vi "Gamepad NanoDrive Control.vi"(1 "handle":i32) -> ()   [LabVIEW 2012]
uses:
  <vilib>/Utility/miscctls.llb/LVPointTypeDef.ctl
  <vilib>/Utility/file.llb/Read From Spreadsheet File (I64).vi
  <vilib>/Utility/inputDevices.llb/joystickAcquire.vi
  <vilib>/Utility/inputDevices.llb/closeJoystick.vi
  Madlib.dll
panel:
  out "Y axis":dbl
  out "X axis":dbl
  out "yRead":dbl=5.0 step=0.1 format="%.3f"
  out "xRead":dbl=5.0 step=0.1 format="%.3f"
  in  "left":bool
  in  "down":bool
  in  "right":bool
  in  "up":bool
  in  "closed?":bool
  in  "Slide":cluster{u32, u32}(slide)={0, 5} scale=0.0..7.0
  in  "configure":bool
  out "button selection refs":T1
  in  "yf":u16(ring)=4 items=["1 X"=1, "2 A"=2, "3 B"=3, "4 Y"=4, "5 LB"=5, "6 RB"=6, "7 LT"=7, "8 RT"=8, "9 Back"=9]
  in  "xf":u16(ring)=3 items=["1 X"=1, "2 A"=2, "3 B"=3, "4 Y"=4, "5 LB"=5, "6 RB"=6, "7 LT"=7, "8 RT"=8, "9 Back"=9]
  in  "yf xr 2":u16(ring)=5 items=["1 X"=1, "2 A"=2, "3 B"=3, "4 Y"=4, "5 LB"=5, "6 RB"=6, "7 LT"=7, "8 RT"=8, "9 Back"=9]
  in  "halt 3":u16(ring)=9 items=["1 X"=1, "2 A"=2, "3 B"=3, "4 Y"=4, "5 LB"=5, "6 RB"=6, "7 LT"=7, "8 RT"=8, "9 Back"=9]
  in  "yf xf 2":u16(ring)=6 items=["1 X"=1, "2 A"=2, "3 B"=3, "4 Y"=4, "5 LB"=5, "6 RB"=6, "7 LT"=7, "8 RT"=8, "9 Back"=9]
  in  "yr xr 2":u16(ring)=7 items=["1 X"=1, "2 A"=2, "3 B"=3, "4 Y"=4, "5 LB"=5, "6 RB"=6, "7 LT"=7, "8 RT"=8, "9 Back"=9]
  in  "yr":u16(ring)=2 items=["1 X"=1, "2 A"=2, "3 B"=3, "4 Y"=4, "5 LB"=5, "6 RB"=6, "7 LT"=7, "8 RT"=8, "9 Back"=9]
  in  "yr xf 2":u16(ring)=8 items=["1 X"=1, "2 A"=2, "3 B"=3, "4 Y"=4, "5 LB"=5, "6 RB"=6, "7 LT"=7, "8 RT"=8, "9 Back"=9]
  in  "xr":u16(ring)=1 items=["1 X"=1, "2 A"=2, "3 B"=3, "4 Y"=4, "5 LB"=5, "6 RB"=6, "7 LT"=7, "8 RT"=8, "9 Back"=9]
  in  "down-left":bool
  in  "down-right":bool
  in  "up-left":bool
  in  "up-right":bool
  in  "yStep":dbl=1.0 min=0.01905 max=4.0 format="%.3f"
  in  "xStep":dbl=1.0 min=0.01905 max=4.0 format="%.3f"
  in  "Invert":bool=TRUE
  in  "Invert":bool
  # "Single Step Controls"
  # "Position"
  # "Step distance"
  # "Current position"
  # "X axis"
  # "X axis"
  # "um"
  # "um"
  # "Y axis"
  # "Y axis"
  # "um"
  # "um"
  # "Step"
  # "Commanded position"
  # "um"
  # "um"
  # "Configuration"
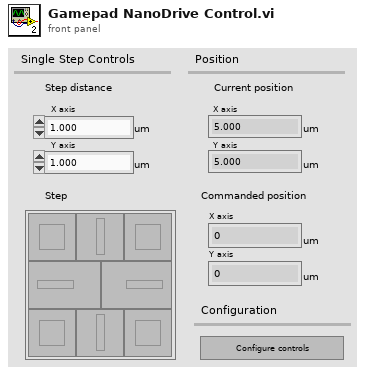
[diagram p1: front panel]
types:
  T1 = cluster{"xr":refnum<vi>, "yr":refnum<vi>, "xf":refnum<vi>, "yf":refnum<vi>, "yf xr 2":refnum<vi>, "yf xf 2":refnum<vi>, "yr xr 2":refnum<vi>, "yr xf 2":refnum<vi>, "halt 2":refnum<vi>}
  T2 = enum16{"open", "replace", "create", "open or create", "replace or create", "replace or create with confirmation"}
  T3 = typedef "LVPointTypeDef.ctl" = cluster{"Horizontal":i16, "Vertical":i16}
  T4 = cluster{"Controls":cluster{"Commands":cluster{"unused":bool}, "Values":cluster{"up":u16, "right":u16}}, "ControlRefs":cluster{"Commands":cluster{"unused":refnum<vi>}, "Values":cluster{"up":refnum<vi>, "right":refnum<vi>}}, "Variables":cluster{"Commands":cluster{"up_changed":bool, "right_changed":bool}, "Values":cluster{"unused":i32}}}
  T5 = cluster{"Controls":cluster{"Commands":cluster{"right":bool, "left":bool, "up":bool, "down":bool, "down-left":bool, "up-left":bool, "up-right":bool, "down-right":bool}, "Values":cluster{"xStep":dbl, "yStep":dbl, "xRead":dbl, "yRead":dbl}}, "ControlRefs":cluster{"Commands":cluster{"right":refnum<vi>, "left":refnum<vi>, "up":refnum<vi>, "down":refnum<vi>, "down-left":refnum<vi>, "up-left":refnum<vi>, "up-right":refnum<vi>, "down-right":refnum<vi>}, "Values":cluster{"X step":refnum<vi>, "Y step":refnum<vi>, "xRead":refnum<vi>, "yRead":refnum<vi>}}, "Variables":cluster{"Commands":cluster{"unused":bool}, "Values":cluster{"xCommand":dbl, "yCommand":dbl, "xCalibration":dbl, "yCalibration":dbl}}}
  T6 = cluster{"xr":refnum<vi>, "yr":refnum<vi>, "xf":refnum<vi>, "yf":refnum<vi>, "yf xr 2":refnum<vi>, "yf xf 2":refnum<vi>, "yr xr 2":refnum<vi>, "yr xf 2":refnum<vi>, "halt 3":refnum<vi>}
  T7 = cluster{"X axis":i32, "Y axis":i32, "Z axis":i32, "X axis rotation":i32, "Y axis rotation":i32, "Z axis rotation":i32, "U axis":i32, "V axis":i32}
  T8 = cluster{"button 1":bool, "button 2":bool, "button 3":bool, "button 4":bool, "button 5":bool, "button 6":bool, "button 7":bool, "button 8":bool, "button 9":bool, "button 10":bool, "button 11":bool, "button 12":bool, "button 13":bool, "button 14":bool, "button 15":bool, "button 16":bool, "button 17":bool, "button 18":bool, "button 19":bool, "button 20":bool, "button 21":bool, "button 22":bool, "button 23":bool, "button 24":bool, "button 25":bool, "button 26":bool, "button 27":bool, "button 28":bool, "button 29":bool, "button 30":bool, "button 31":bool, "button 32":bool}
  T9 = cluster{"left":bool, "down":bool, "right":bool, "up":bool, "up-left":bool, "up-right":bool, "down-left":bool, "down-right":bool, "halt":bool, "button 10":bool}
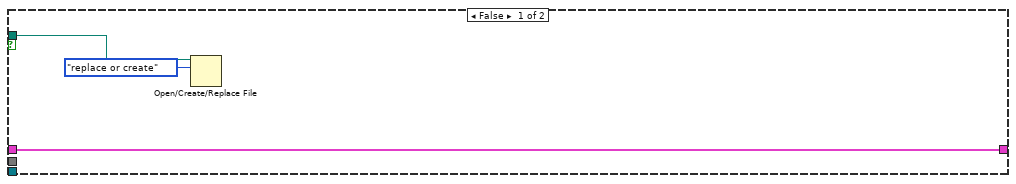
[diagram p2: hidden frame]
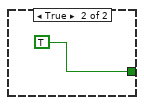
[diagram p4: hidden frame]
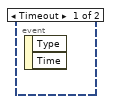
[diagram p9: hidden frame]
diagram:
  n1 = flat-sequence {
    tunnel: [w54] -> w39
    tunnel: [w53] -> w38
    tunnel: [w52] -> w37
    tunnel: [w71] -> w32
    tunnel: [w70] -> w31
    tunnel: [w69] -> w30
    tunnel: w39 -> [w71]
    tunnel: w38 -> [w66]
    tunnel: w37 -> [w69]
    tunnel: w32 -> [w74]
    tunnel: [w73] -> w41
    tunnel: w31 -> [w84]
    tunnel: [w84] -> w40
    tunnel: w30 -> [w72]
    tunnel: [w72] -> w36
    tunnel: w41 -> [w90]
    tunnel: [w90] -> w43
    tunnel: w40 -> [w96]
    tunnel: [w96] -> w42
    tunnel: w36 -> [w87]
    tunnel: [w86] -> w34
    tunnel: [w145] -> w47
    tunnel: [w146] -> w45
    tunnel: w42 -> [w146]
    tunnel: w43 -> [w145]
    tunnel: [w138] -> w35
    tunnel: w34 -> [w138]
    tunnel: [w151] -> w15
    tunnel: [w150] -> w13
    tunnel: w47 -> [w149]
    tunnel: [w149] -> w11
    tunnel: [w148] -> w9
    tunnel: w45 -> [w148]
    tunnel: [w147] -> w7
    tunnel: w35 -> [w147]
    tunnel: w15 -> [w176]
    tunnel: [w176] -> w14
    tunnel: w13 -> [w175]
    tunnel: [w175] -> w12
    tunnel: w11 -> [w174]
    tunnel: [w174] -> w10
    tunnel: w9 -> [w173]
    tunnel: [w173] -> w8
    tunnel: w7 -> [w172]
    tunnel: [w172] -> w6
    tunnel: ["handle"] -> w5
    tunnel: [w183] -> w27
    tunnel: [w184] -> w25
    tunnel: [w182] -> w23
    tunnel: w14 -> [w184]
    tunnel: w12 -> [w183]
    tunnel: w10 -> [w181]
    tunnel: [w181] -> w21
    tunnel: w8 -> [w180]
    tunnel: [w180] -> w19
    tunnel: w6 -> [w179]
    tunnel: [w179] -> w17
    tunnel: w5 -> [w178]
    tunnel: [w177] -> w4
    tunnel: w27 -> [w211]
    tunnel: [w211] -> w26
    tunnel: w25 -> [w210]
    tunnel: [w210] -> w24
    tunnel: w23 -> [w206]
    tunnel: [w206] -> w22
    tunnel: w21 -> [w205]
    tunnel: [w205] -> w20
    tunnel: w19 -> [w204]
    tunnel: [w201] -> w18
    tunnel: w17 -> [w209]
    tunnel: [w209] -> w16
    tunnel: w4 -> [w200]
    tunnel: [w200] -> w2
    tunnel: w26 -> [w219]
    tunnel: [w219] -> w51
    tunnel: w24 -> [w220]
    tunnel: [w220] -> w50
    tunnel: w22 -> [w218]
    tunnel: [w218] -> w49
    tunnel: [u32 0 ("current button state")] -> w48
    tunnel: [w215] -> w46
    tunnel: w20 -> [w215]
    tunnel: [w214] -> w44
    tunnel: w18 -> [w214]
    tunnel: [w213] -> w33
    tunnel: w16 -> [w213]
    tunnel: [w212] -> w3
    tunnel: w2 -> [w212]
    tunnel: w49 -> [w229]
    tunnel: w50 -> [w231]
    tunnel: w51 -> [w230]
    tunnel: w48 -> [w228]
    tunnel: w46 -> [w227]
    tunnel: w44 -> [w226]
    tunnel: w33 -> [w225]
    tunnel: [w224] -> w29
    tunnel: [w223] -> w28
    tunnel: w3 -> [w222]
    tunnel: [w221] -> w1
    tunnel: w29 -> [_]
    tunnel: w28 -> [w542]
    tunnel: w1 -> [_]
    frame #0 {
      w52 = T4 {"Controls"={"Commands"={"unused"=FALSE}, "Values"={"up"=2, "right"=0}}, "ControlRefs"={"Commands"={"unused"=refnum}, "Values"={"up"=refnum, "right"=refnum}}, "Variables"={"Commands"={"up_changed"=FALSE, "right_changed"=FALSE}, "Values"={"unused"=0}}}  # Configuration
      w53 = T5 {"Controls"={"Commands"={"right"=FALSE, "left"=FALSE, "up"=FALSE, "down"=FALSE, "down-left"=FALSE, "up-left"=FALSE, "up-right"=FALSE, "down-right"=FALSE}, "Values"={"xStep"=1.0, "yStep"=1.0, "xRead"=1.0, "yRead"=1.0}}, "ControlRefs"={"Commands"={"right"=refnum, "left"=refnum, "up"=refnum, "down"=refnum, "down-left"=refnum, "up-left"=refnum, "up-right"=refnum, "down-right"=refnum}, "Values"={"X step"=refnum, "Y step"=refnum, "xRead"=refnum, "yRead"=refnum}}, "Variables"={"Commands"={"unused"=FALSE}, "Values"={"xCommand"=0.0, "yCommand"=0.0, "xCalibration"=0.0, "yCalibration"=0.0}}}  # Motion
      w54 = T6 {"xr"=refnum, "yr"=refnum, "xf"=refnum, "yf"=refnum, "yf xr 2"=refnum, "yf xf 2"=refnum, "yr xr 2"=refnum, "yr xf 2"=refnum, "halt 3"=refnum}  # output cluster
    }
    frame #1 {
      n2 = control-ref of="right"() -> (w64:refnum<vi>)
      n3 = control-ref of="left"() -> (w63:refnum<vi>)
      n4 = control-ref of="up"() -> (w62:refnum<vi>)
      n5 = control-ref of="down"() -> (w61:refnum<vi>)
      n6 = control-ref of="down-left"() -> (w60:refnum<vi>)
      n7 = control-ref of="up-left"() -> (w59:refnum<vi>)
      n8 = control-ref of="up-right"() -> (w58:refnum<vi>)
      n9 = control-ref of="down-right"() -> (w57:refnum<vi>)
      n10 = control-ref of="xStep"() -> (w67:refnum<vi>)
      n11 = control-ref of="yStep"() -> (w68:refnum<vi>)
      n12 = control-ref of="xRead"() -> (w56:refnum<vi>)
      n13 = control-ref of="yRead"() -> (w55:refnum<vi>)
      n14 = Bundle By Name(cluster=w66, "ControlRefs.Values.X step"=w67, "ControlRefs.Values.Y step"=w68, "ControlRefs.Values.xRead"=w56, "ControlRefs.Values.yRead"=w55) -> (w65:T5)
      n15 = Bundle By Name(cluster=w65, "ControlRefs.Commands.right"=w64, "ControlRefs.Commands.left"=w63, "ControlRefs.Commands.up"=w62, "ControlRefs.Commands.down"=w61, "ControlRefs.Commands.down-left"=w60, "ControlRefs.Commands.up-left"=w59, "ControlRefs.Commands.up-right"=w58, "ControlRefs.Commands.down-right"=w57) -> (w70:T5)
    }
    frame #2 {
      n16 = control-ref of="xr"() -> (w83:refnum<vi>)
      n17 = control-ref of="yr"() -> (w82:refnum<vi>)
      n18 = control-ref of="xf"() -> (w81:refnum<vi>)
      n19 = control-ref of="yf"() -> (w80:refnum<vi>)
      n20 = control-ref of="yf xr 2"() -> (w79:refnum<vi>)
      n21 = control-ref of="yf xf 2"() -> (w78:refnum<vi>)
      n22 = control-ref of="yr xr 2"() -> (w77:refnum<vi>)
      n23 = control-ref of="yr xf 2"() -> (w76:refnum<vi>)
      n24 = control-ref of="halt 3"() -> (w75:refnum<vi>)
      n25 = Bundle(cluster=w74, "xr"=w83, "yr"=w82, "xf"=w81, "yf"=w80, "yf xr 2"=w79, "yf xf 2"=w78, "yr xr 2"=w77, "yr xf 2"=w76, "halt 3"=w75) -> (w73:T6)
    }
    frame #3 {
      n26 = control-ref of="This Application"() -> (w95:refnum<vi>)
      n27 = property class="App"(reference=w95) -> ("App.Dir"=w89:path)  [unwired: 1 in, 2 out]
      n28 = control-ref of="Slide"() -> (w92:refnum<vi>)
      n29 = Build Path(base path=w89, name or relative path="config.txt") -> (appended path=w93:path)
      n30 = Cluster To Array(cluster=w90) -> (array=w91:refnum<vi>[])
      n31 = call <vilib>:"Check if File or Folder Exists.vi"("path"=w93) -> ("file or folder exists?"=w85:bool, "dup path"=w88:path)  [unwired: 1 in, 8 out]
      n32 = case shown="True" w85 {
        tunnel: w92 -> [_ w113]
        tunnel: w91 -> [_ w112]
        tunnel: w88 -> [w99 w111]
        tunnel: w87 -> [w97 w101]
        tunnel: [w97 w100] -> w86
        frame False {
          n33 = Open/Create/Replace File(file path (use dialog)=w99, operation (0:open)=T2."replace or create") -> ()  [unwired: 1 in, 6 out]
        }
        frame True {
          n34 = Read from Text File(file (use dialog)=w111) -> (text=w110:string)  [unwired: 1 in, 5 out]
          n35 = String To Path(string=w110) -> (path=w109:path)
          n36 = call <vilib>:"Check if File or Folder Exists.vi"("path"=w109) -> ("file or folder exists?"=w107:bool, "dup path"=w103:path)  [unwired: 1 in, 8 out]
          n37 = Not A Number/Path/Refnum?(number/path/refnum=w103) -> (NaN/Path/Refnum?=w106:bool)
          n38 = Empty String/Path?(string/path=w103) -> (empty?=w104:bool)
          n39 = Not(x=w106) -> (.not. x?=w105:bool)
          n40 = Not(x=w104) -> (.not. x?=w102:bool)
          n41 = Compound Arithmetic op=AND(w105, w107, w102) -> (w108:bool)
          n42 = case shown="True" w108 {
            tunnel: w112 -> [_ w132]
            tunnel: w113 -> [_ w133]
            tunnel: w103 -> [_ w131]
            tunnel: w101 -> [w114 w130]
            tunnel: [w114 w129] -> w100
            frame False {
            }
            frame True {
              n43 = call-poly <vilib>:"Read From Spreadsheet File.vi"("transpose (no:F)"=TRUE ("transpose? (no:F)"), "file path (dialog if empty)"=w131) -> ("first row"=w134:i64[])  [unwired: 2 in, 7 out]
              n44 = Array Size(array=w132) -> (size(s)=w128:i32)
              n45 = Split 1D Array(array=w134, index=w128) -> (first subarray=w125:i64[], second subarray=w127:i64[])
              n46 = Index Array(array=w127) -> (element #1=w117:i64, element #2=w118:i64, element #3=w124:i64, element #4=w121:i64, element #5=w116:i64, element #6=w115:i64)  [unwired: 6 in]
              n47 = Bundle(w118, w117) -> (w126:cluster{i64, i64})  [unwired: 1 out]
              n48 = property class="Slide (strict)"(reference=w133, "Value"=w126) -> ()  [unwired: 1 in, 2 out]
              n49 = Bundle By Name(cluster=w130, "Controls.Values.up"=w116, "Controls.Values.right"=w115) -> (w129:T4)
              n50 = control-ref of="Invert"() -> (w120:refnum<vi>)
              n51 = control-ref of="Invert"() -> (w119:refnum<vi>)
              n52 = Greater Than 0?(x=w124) -> (x > 0?=w123:bool)
              n53 = Greater Than 0?(x=w121) -> (x > 0?=w122:bool)
              n54 = property class="Bool (strict)"(reference=w120, "Value"=w123) -> ()  [unwired: 1 in, 2 out]
              n55 = property class="Bool (strict)"(reference=w119, "Value"=w122) -> ()  [unwired: 1 in, 2 out]
              n56 = for {
                tunnel: w132 -> [w137] mode=indexing
                tunnel: w125 -> [w136] mode=indexing
                n57 = property class="Ring (strict)"(reference=w137, "Value"=w136) -> ()  [unwired: 1 in, 2 out]
              }
            }
          }
        }
      }
    }
    frame #4 {
      w141 = TRUE ("Front Panel Window:Closeable")
      w142 = FALSE ("Front Panel Window:Title Bar Visible")
      n58 = control-ref of="Pane"() -> (w139:refnum<vi>)
      n59 = control-ref of="This VI"() -> (w144:refnum<vi>)
      n60 = property class="VI"(reference=w144, "Front Panel.Title"="Gamepad NanoDrive Control" ("Front Panel Window:Title"), "Front Panel.TitleBarVis"=w141, "TB.Visible"=w142, "Front Panel.ShowMenuBar"=w142, "Front Panel.Closeable"=w141) -> ()  [unwired: 1 in, 2 out]
      n61 = property class="Pane"(reference=w139, "Origin"=T3 {"Horizontal"=0, "Vertical"=0}) -> ()  [unwired: 1 in, 2 out]
    }
    frame #5 {
      n62 = while {
        tunnel: [w157] -> w150
        tunnel: [w152] -> w151
        stop <- w156 stop-if-true
        n63 = flat-sequence {
          tunnel: [w160] -> w159
          tunnel: [w161] -> w158
          tunnel: [w160] -> w155
          tunnel: w159 -> [w165]
          tunnel: [w164] -> w157
          tunnel: w158 -> [w164]
          tunnel: [w163] -> w152
          tunnel: w155 -> [w163]
          tunnel: [w162] -> w154
          frame #0 {
            n64 = call "init joystick.vi"() -> ("device ID"=w161:refnum<k1>, "Joystick found"=w160:bool)  [unwired: 2 out]
          }
          frame #1 {
            n65 = case shown="False" w165 {
              tunnel: [w166 TRUE ("T button?")] -> w162
              frame False {
                n66 = Two Button Dialog(message="Press start (button 10)\n on your Gamepad \n(while pressing 'Ok')\nfor it to be initialized. ", 1:"Cancel Program" ("F button name (\"Cancel\")"), 2:"Ok" ("T button name (\"OK\")")) -> (T button?=w166:bool)
              }
              frame True {
              }
            }
          }
        }
        n67 = Not(x=w154) -> (.not. x?=w153:bool)
        n68 = Or(x=w153, y=w152) -> (x .or. y?=w156:bool)
      }
    }
    frame #6 {
    }
    frame #7 {
      n69 = Less Or Equal To 0?(x=w178) -> (x <= 0?=w177:bool)
      n70 = case shown="True" w177 {
        tunnel: [w185 w186] -> w182
        tunnel: w178 -> [w185 _]
        frame False {
        }
        frame True {
          n71 = dll-call lib="C:/Users/Labview/Desktop/64-bit VIs/Madlib.dll" fn="MCL_InitHandleOrGetExisting"() -> ("return type"=w187:i32)  [unwired: 3 in, 2 out]
          n72 = Less Or Equal To 0?(x=w187) -> (x <= 0?=w188:bool)
          n73 = case shown="True" w188 {
            tunnel: w187 -> [w189 w191]
            tunnel: [w189 w190] -> w186
            frame False {
            }
            frame True {
              n74 = while {
                tunnel: w191 -> [w196]
                tunnel: [w194] -> w190
                stop <- w193 continue-if-true
                n75 = Two Button Dialog(message="Failed to load NanoDrive!\nReInit?") -> (T button?=w192:bool)  [unwired: 2 out]
                n76 = case shown="True" w192 {
                  tunnel: w196 -> [w198 _]
                  tunnel: [w198 w199] -> w194
                  frame False {
                  }
                  frame True {
                    n77 = dll-call lib="C:/Users/Labview/Desktop/64-bit VIs/Madlib.dll" fn="MCL_InitHandleOrGetExisting"() -> ("return type"=w199:i32)  [unwired: 3 in, 2 out]
                  }
                }
                n78 = Less Or Equal To 0?(x=w194) -> (x <= 0?=w195:bool)
                n79 = And(x=w192, y=w195) -> (x .and. y?=w193:bool)
              }
            }
          }
        }
      }
    }
    frame #8 {
      n80 = dll-call lib="C:/Users/Labview/Desktop/64-bit VIs/Madlib.dll" fn="MCL_GetCalibration" ("MADLib.dll:MCL_InitHandleOrGetExisting")("axis"=1, "handle"=w206) -> ("calibration"=w203:dbl)  [unwired: 3 in, 4 out]
      n81 = dll-call lib="C:/Users/Labview/Desktop/64-bit VIs/Madlib.dll" fn="MCL_GetCalibration" ("MADLib.dll:MCL_InitHandleOrGetExisting")("axis"=2, "handle"=w206) -> ("calibration"=w202:dbl)  [unwired: 3 in, 4 out]
      n82 = Bundle By Name(cluster=w204, "Variables.Values.xCalibration"=w203, "Variables.Values.yCalibration"=w202) -> (w201:T5)
    }
    frame #9 {
      n83 = local write "closed?"(FALSE ("closed?")) -> ()
    }
    frame #10 {
      n84 = case shown="True" w231 {
        tunnel: w230 -> [_ w242]
        tunnel: w229 -> [_ w241]
        tunnel: w228 -> [_ w240]
        tunnel: w227 -> [_ w239]
        tunnel: w226 -> [_ w235]
        tunnel: w225 -> [_ w238]
        tunnel: [_ w237] -> w224
        tunnel: [_ w236] -> w223
        tunnel: w222 -> [_ w234]
        tunnel: [_ w233] -> w221
        frame False {
        }
        frame True {
          n85 = while {
            tunnel: w242 -> [w354]
            tunnel: [w353] -> w236
            tunnel: [w352] -> w237
            tunnel: w241 -> [w351]
            shift-right: [w350] -> _
            shift-left: w240 -> [w349]
            tunnel: w239 -> [w341]
            shift-right: [w320] -> _
            shift-left: w238 -> [w325]
            shift-right: [w307] -> _
            shift-left: w235 -> [w306]
            tunnel: w234 -> [w257]
            tunnel: [w245] -> w233
            stop <- w348 stop-if-true
            n86 = Wait Until Next ms Multiple(millisecond multiple=u32 10) -> ()  [unwired: 1 out]
            n87 = flat-sequence {
              tunnel: [w370] -> w319
              tunnel: [w369] -> w318
              tunnel: [w368] -> w317
              tunnel: [w367] -> w316
              tunnel: [w366] -> w315
              tunnel: [w365] -> w314
              tunnel: w349 -> [w370]
              tunnel: w351 -> [w369]
              tunnel: w354 -> [w368]
              tunnel: w341 -> [w367]
              tunnel: w325 -> [w365]
              tunnel: w306 -> [w356]
              tunnel: [w355] -> w258
              tunnel: w257 -> [w355]
              tunnel: [w380] -> w313
              tunnel: [w379] -> w312
              tunnel: [w378] -> w311
              tunnel: [w375] -> w310
              tunnel: [w377] -> w309
              tunnel: [w376] -> w308
              tunnel: w314 -> [w376]
              tunnel: w315 -> [w374]
              tunnel: w316 -> [w375]
              tunnel: w317 -> [w378]
              tunnel: w318 -> [w379]
              tunnel: w319 -> [w380]
              tunnel: w258 -> [w371]
              tunnel: [w371] -> w254
              tunnel: [w391] -> w347
              tunnel: [w390] -> w345
              tunnel: [w389] -> w343
              tunnel: [w388] -> w339
              tunnel: w313 -> [w391]
              tunnel: w312 -> [w390]
              tunnel: w311 -> [w389]
              tunnel: w310 -> [w388]
              tunnel: [w384] -> w332
              tunnel: w309 -> [w384]
              tunnel: w308 -> [w387]
              tunnel: [w387] -> w323
              tunnel: [w381] -> w255
              tunnel: w254 -> [w381]
              tunnel: w347 -> [w400]
              tunnel: [w400] -> w346
              tunnel: w345 -> [w399]
              tunnel: [w399] -> w344
              tunnel: w343 -> [w397]
              tunnel: [w397] -> w342
              tunnel: [w396] -> w340
              tunnel: w339 -> [w396]
              tunnel: [w395] -> w333
              tunnel: w332 -> [w395]
              tunnel: [w393] -> w324
              tunnel: w323 -> [w394]
              tunnel: [w392] -> w256
              tunnel: w255 -> [w392]
              tunnel: [w420] -> w330
              tunnel: [w413] -> w329
              tunnel: [w419] -> w328
              tunnel: [w418] -> w327
              tunnel: [w415] -> w326
              tunnel: [w417] -> w322
              tunnel: w324 -> [w417]
              tunnel: w333 -> [w416]
              tunnel: w340 -> [w418]
              tunnel: w342 -> [w420]
              tunnel: w344 -> [w413]
              tunnel: w346 -> [w419]
              tunnel: w256 -> [w409]
              tunnel: [w409] -> w251
              tunnel: [w429] -> w338
              tunnel: [w428] -> w337
              tunnel: [w427] -> w336
              tunnel: [w423] -> w335
              tunnel: [w426] -> w334
              tunnel: [w425] -> w331
              tunnel: [w424] -> w321
              tunnel: [w422] -> w295
              tunnel: w330 -> [w429]
              tunnel: w329 -> [w428]
              tunnel: w328 -> [w427]
              tunnel: w327 -> [w422]
              tunnel: w326 -> [w425]
              tunnel: w322 -> [w424]
              tunnel: [w421] -> w252
              tunnel: w251 -> [w421]
              tunnel: [w463] -> w301
              tunnel: [w464] -> w302
              tunnel: [w462] -> w303
              tunnel: [w461] -> w304
              tunnel: [w460] -> w305
              tunnel: [w459] -> w300
              tunnel: [w458] -> w299
              tunnel: [w457] -> w298
              tunnel: w321 -> [w460]
              tunnel: w331 -> [w461]
              tunnel: w334 -> [w432]
              tunnel: w335 -> [w459]
              tunnel: w336 -> [w462]
              tunnel: w337 -> [w464]
              tunnel: w338 -> [w463]
              tunnel: [w431] -> w296
              tunnel: w295 -> [w431]
              tunnel: [w430] -> w253
              tunnel: w252 -> [w430]
              tunnel: [w475] -> w284
              tunnel: [w476] -> w286
              tunnel: [w478] -> w288
              tunnel: [w472] -> w290
              tunnel: [w477] -> w292
              tunnel: [w474] -> w294
              tunnel: [w473] -> w282
              tunnel: [w471] -> w276
              tunnel: [w470] -> w275
              tunnel: w296 -> [w473]
              tunnel: w298 -> [w469]
              tunnel: w299 -> [w468]
              tunnel: w300 -> [w474]
              tunnel: w301 -> [w475]
              tunnel: w302 -> [w476]
              tunnel: w303 -> [w478]
              tunnel: w304 -> [w472]
              tunnel: w305 -> [w477]
              tunnel: w253 -> [w465]
              tunnel: [w465] -> w248
              tunnel: w294 -> [w485]
              tunnel: [w483] -> w293
              tunnel: w292 -> [w490]
              tunnel: [w490] -> w291
              tunnel: w290 -> [w489]
              tunnel: [w489] -> w289
              tunnel: w288 -> [w484]
              tunnel: [w479] -> w287
              tunnel: w286 -> [w488]
              tunnel: [w488] -> w285
              tunnel: w284 -> [w487]
              tunnel: [w487] -> w283
              tunnel: w282 -> [w486]
              tunnel: w276 -> [w481]
              tunnel: w275 -> [w482]
              tunnel: [w482] -> w274
              tunnel: [w481] -> w273
              tunnel: [w480] -> w249
              tunnel: w248 -> [w480]
              tunnel: [w503] -> w264
              tunnel: [w496] -> w266
              tunnel: [w502] -> w268
              tunnel: [w501] -> w270
              tunnel: [w500] -> w272
              tunnel: w293 -> [w497]
              tunnel: w291 -> [w500]
              tunnel: w289 -> [w501]
              tunnel: w287 -> [w502]
              tunnel: w285 -> [w496]
              tunnel: w283 -> [w503]
              tunnel: [w495] -> w262
              tunnel: w274 -> [w495]
              tunnel: [w494] -> w261
              tunnel: w273 -> [w494]
              tunnel: [w493] -> w260
              tunnel: [w492] -> w259
              tunnel: [w491] -> w250
              tunnel: w249 -> [w491]
              tunnel: w272 -> [w524]
              tunnel: [w524] -> w271
              tunnel: w270 -> [w510]
              tunnel: [w509] -> w269
              tunnel: w268 -> [w523]
              tunnel: [w523] -> w267
              tunnel: w266 -> [w522]
              tunnel: [w522] -> w265
              tunnel: w264 -> [w521]
              tunnel: [w521] -> w263
              tunnel: w262 -> [w508]
              tunnel: w261 -> [w507]
              tunnel: w260 -> [w506]
              tunnel: w259 -> [w505]
              tunnel: w250 -> [w504]
              tunnel: [w504] -> w246
              tunnel: w271 -> [w534]
              tunnel: [w534] -> w281
              tunnel: w269 -> [w528]
              tunnel: [w528] -> w280
              tunnel: w267 -> [w533]
              tunnel: [w533] -> w279
              tunnel: w265 -> [w529]
              tunnel: [w529] -> w278
              tunnel: w263 -> [w532]
              tunnel: [w532] -> w277
              tunnel: [w525] -> w247
              tunnel: w246 -> [w525]
              tunnel: [w539] -> w350
              tunnel: [w540] -> w352
              tunnel: [w541] -> w353
              tunnel: ["closed?"] -> w348
              tunnel: [w537] -> w320
              tunnel: w281 -> [w537]
              tunnel: w280 -> [w536]
              tunnel: w279 -> [w539]
              tunnel: w278 -> [w540]
              tunnel: w277 -> [w541]
              tunnel: [w536] -> w307
              tunnel: w247 -> [w535]
              tunnel: [w535] -> w245
              frame #0 {
                # "Update control values"
                n88 = Bundle By Name(cluster=w356, "Controls.Commands.right"="right", "Controls.Commands.left"="left", "Controls.Commands.up"="up", "Controls.Commands.down"="down", "Controls.Commands.down-left"="down-left", "Controls.Commands.up-left"="up-left", "Controls.Commands.up-right"="up-right", "Controls.Commands.down-right"="down-right") -> (w366:T5)
              }
              frame #1 {
                # "Update control values"
                n89 = Bundle By Name(cluster=w374, "Controls.Values.xStep"="xStep", "Controls.Values.yStep"="yStep") -> (w377:T5)
              }
              frame #2 {
                # "Display device info"
                n90 = Unbundle By Name(w384) -> ("Variables.Values.xCommand"=→"X axis":dbl, "Variables.Values.yCommand"=→"Y axis":dbl)
                n91 = Unbundle By Name(w384) -> ("Controls.Values.xRead"=→"xRead":dbl, "Controls.Values.yRead"=→"yRead":dbl)
              }
              frame #3 {
                # "Configure the Gamepad control stick and buttons."
                n92 = case shown="True" "configure" {
                  tunnel: w397 -> [_ w405]
                  tunnel: w396 -> [_ w404]
                  tunnel: w394 -> [w401 w403]
                  tunnel: [w401 w402] -> w393
                  frame False {
                  }
                  frame True {
                    n93 = control-ref of="Invert"() -> (w407:refnum<vi>)
                    n94 = control-ref of="Invert"() -> (w406:refnum<vi>)
                    n95 = control-ref of="Slide"() -> (w408:refnum<vi>)
                    n96 = call "Configure Gamepad.vi"("Cluster"=w404, "Configuration"=w403, "Slide 2"=w408, "invert y"=w406, "invert x"=w407, "device ID"=w405) -> ("Configuration"=w402:T4)  [unwired: 5 out]
                  }
                }
              }
              frame #4 {
                # "Read the ADCs"
                n97 = dll-call lib="C:/Users/Labview/Desktop/64-bit VIs/Madlib.dll" fn="MCL_SingleReadN"("axis"=1, "handle"=w413) -> ("position"=w411:dbl)  [unwired: 4 in, 3 out]
                n98 = dll-call lib="C:/Users/Labview/Desktop/64-bit VIs/Madlib.dll" fn="MCL_SingleReadN"("axis"=2, "handle"=w413) -> ("position"=w410:dbl)  [unwired: 4 in, 3 out]
                n99 = Bundle By Name(cluster=w416, "Controls.Values.xRead"=w411, "Controls.Values.yRead"=w410) -> (w415:T5)
              }
              frame #5 {
                # "Get the Gamepad info"
                n100 = call-poly <vilib>:"Acquire Input Data.vi"("device ID"=w429) -> ("axis info"=w426:T7, "button info"=w423:T8)  [unwired: 1 in, 16 out]
              }
              frame #6 {
                w454 = 0.05 ("return type")
                w455 = 0.05 ("return type")
                # "Get a number from -1 to 1 representing the control-stick position"
                n101 = Cluster To Array(cluster=w432) -> (array=w437:i32[])
                n102 = Unbundle("Slide") -> (w435:u32, w434:u32)
                n103 = Index Array(array=w437, index #1=w435, index #2=w434) -> (element #1=w438:i32, element #2=w433:i32)
                n104 = Negate(x=w433) -> (-x=w440:i32)
                n105 = Negate(x=w438) -> (-x=w450:i32)
                n106 = Select(t=w440, s="Invert", f=w433) -> (s? t:f=w452:i32)
                n107 = Select(t=w450, s="Invert", f=w438) -> (s? t:f=w451:i32)
                n108 = Divide(x=w451, y=32768) -> (x/y=w442:dbl)
                n109 = Negate(x=w455) -> (-x=w456:dbl)
                n110 = Divide(x=w452, y=32768) -> (x/y=w441:dbl)
                n111 = Negate(x=w454) -> (-x=w453:dbl)
                n112 = In Range and Coerce(upper limit=w455, x=w441, lower limit=w456) -> (In Range?=w446:bool)  [unwired: 1 out]
                n113 = In Range and Coerce(upper limit=w454, x=w442, lower limit=w453) -> (In Range?=w444:bool)  [unwired: 1 out]
                n114 = Select(t=0.0, s=w444, f=w442) -> (s? t:f=w457:dbl)
                n115 = Select(t=0.0, s=w446, f=w441) -> (s? t:f=w458:dbl)
              }
              frame #7 {
                # "Change the -1 to 1 control-stick value to something much smaller"
                n116 = Divide(x=w469, y=100.0) -> (x/y=w471:dbl)
                n117 = Divide(x=w468, y=100.0) -> (x/y=w470:dbl)
              }
              frame #8 {
                # "Have any Gamepad buttons been pressed?"
                n118 = call "user maped buttons.vi"("previous button state"=w484, "gp button info"=w485, "map references"=w486) -> ("current button state"=w479:u32, "mapped gp buttons"=w483:T9)  [unwired: 1 out]
              }
              frame #9 {
                n119 = Unbundle By Name(w501) -> ("Controls.Values.xStep"=w498:dbl, "Controls.Values.yStep"=w499:dbl)
                n120 = call "button commands.vi"("Configuration"=w500, "Motion"=w501, "Y Steps"=w499, "mapped gp buttons"=w497, "X Steps"=w498) -> ("Y distance"=w492:dbl, "X distance"=w493:dbl)  [unwired: 5 out]
              }
              frame #10 {
                n121 = Unbundle By Name(w510) -> ("Variables.Values.xCalibration"=w516:dbl, "Variables.Values.xCommand"=w520:dbl, "Variables.Values.yCommand"=w519:dbl, "Variables.Values.yCalibration"=w512:dbl)
                n122 = Compound Arithmetic op=ADD(w520, w507, w506) -> (w518:dbl)
                n123 = Compound Arithmetic op=ADD(w519, w508, w505) -> (w514:dbl)
                n124 = In Range and Coerce(upper limit=w516, x=w518, lower limit=0.0) -> (coerced(x)=w517:dbl)  [unwired: 1 out]
                n125 = In Range and Coerce(upper limit=w512, x=w514, lower limit=0.0) -> (coerced(x)=w511:dbl)  [unwired: 1 out]
                n126 = Bundle By Name(cluster=w510, "Variables.Values.xCommand"=w517, "Variables.Values.yCommand"=w511) -> (w509:T5)
              }
              frame #11 {
                n127 = Unbundle By Name(w528) -> ("Variables.Values.xCommand"=w527:dbl, "Variables.Values.yCommand"=w526:dbl)
                n128 = dll-call lib="C:/Users/Labview/Desktop/64-bit VIs/Madlib.dll" fn="MCL_SingleWriteN"("command"=w526, "axis"=2, "handle"=w529) -> ()  [unwired: 4 in, 5 out]
                n129 = dll-call lib="C:/Users/Labview/Desktop/64-bit VIs/Madlib.dll" fn="MCL_SingleWriteN"("command"=w527, "axis"=1, "handle"=w529) -> ()  [unwired: 4 in, 5 out]
              }
              frame #12 {
              }
            }
          }
          n130 = event shown="[1] Panel Close?" {
            selector: _ -> [_ _]
            dyn-events: _ -> [_ _]
            timeout: -1 -> [_ _]
            event Timeout {
              n131 = event-data() -> ()  [unwired: 1 in, 2 out]
            }
            event Panel Close? {
              n132 = event-data() -> ()  [unwired: 1 in, 3 out]
              n133 = local write "closed?"(TRUE ("closed?")) -> ()
              n134 = event-data("Discard?"=TRUE) -> ()  [unwired: 1 in, 1 out]
            }
          }
        }
      }
    }
    frame #11 {
      n135 = call-poly <vilib>:"Close Input Device.vi"("device ID"=w542) -> ()  [unwired: 9 in, 1 out]
    }
  }
